vi "Wrap coordiantes off neighbours.vi"(10 "Length":i32, 11 "Index":i32) -> (2 "Translated index":i32)   [LabVIEW 2013]
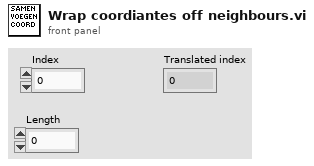
[diagram p1: front panel]
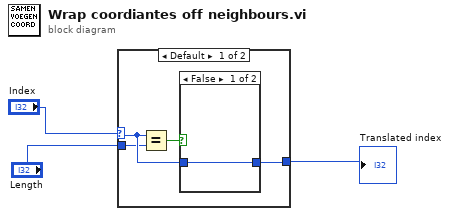
[diagram p0: block diagram]
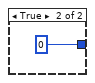
[diagram p2: hidden frame]
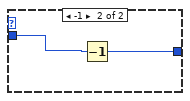
[diagram p3: hidden frame]
diagram:
  n1 = case shown="Default" "Index" {
    selector: "Index" -> [w5 _]
    tunnel: [w6 w11] -> w3
    tunnel: "Length" -> [w4 w10]
    frame Default {
      n2 = Equal?(x=w5, y=w4) -> (x = y?=w7:bool)
      n3 = case shown="False" w7 {
        tunnel: [w8 0 ("Column")] -> w6
        tunnel: w5 -> [w8 _]
        frame False {
        }
        frame True {
        }
      }
    }
    frame -1 {
      n4 = Decrement(x=w10) -> (x-1=w11:i32)
    }
  }
  "Translated index" <- w3
